vi "Add Icon From Path.vi"(7 "Icon Index (Next)":i32=-1, 8 "error in (no error)":errorcluster, 9 "Icon Name":string, 10 "Image Path":path, 11 "Toolbar Control in":refnum<class "Toolbar Control.lvclass">) -> (0 "error out":errorcluster, 3 "Toolbar Control out":refnum<class "Toolbar Control.lvclass">)   [LabVIEW 2011, in "Toolbar Control.lvclass"]
doc: "This VI will add the image <B>Image Path</B> to the <B>Toolbar Control in</B> at the available location or if specified by <B>Icon Index (Next)</B>. The name of the button will default to the file name or one provided by <B>Icon Name</B>. The image file can be a PNG with alpha layers.\n\n-------------\nDeveloped by Brian Hoover (hooovahh)"
uses:
  Toolbar Control.lvclass
  Toolbar Control.lvclass/Toolbar Control.ctl
  Controls/Icon Data.ctl
  <vilib>/picture/picture.llb/imagedata.ctl
  Controls/Button State.ctl
  Controls/Icon Type.ctl
  <vilib>/Utility/miscctls.llb/LVRectTypeDef.ctl
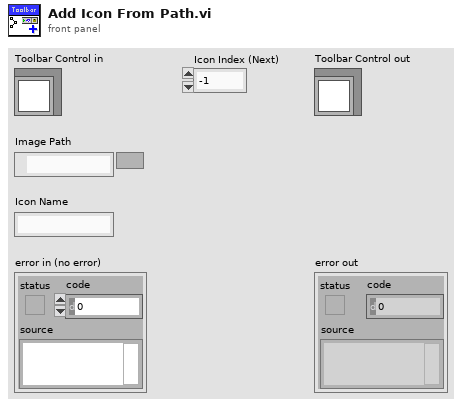
[diagram p1: front panel]
types:
  T1 = typedef "LVRectTypeDef.ctl" = cluster{"Left":i16, "Top":i16, "Right":i16, "Bottom":i16}
  T2 = typedef "Toolbar Control.lvclass/Icon Data.ctl" = cluster{"Original Image Path":path, "Original Image Data":T3, "Scaled Icon":picture, "Button Name":string, "Button State":T4, "Icon Type":T5}
  T3 = typedef "imagedata.ctl" = cluster{"image type":i32, "image depth":i32, "image":u8[], "mask":u8[], "colors":u32[], "Rectangle":cluster{"left":i16, "top":i16, "right":i16, "bottom":i16}}
  T4 = typedef "Toolbar Control.lvclass/Button State.ctl" = enum8{"Enabled", "Disabled", "Disabled and Grayed Out"}
  T5 = typedef "Icon Type.ctl" = enum16{"Normal Icon", "Separator Icon", "More Options"}
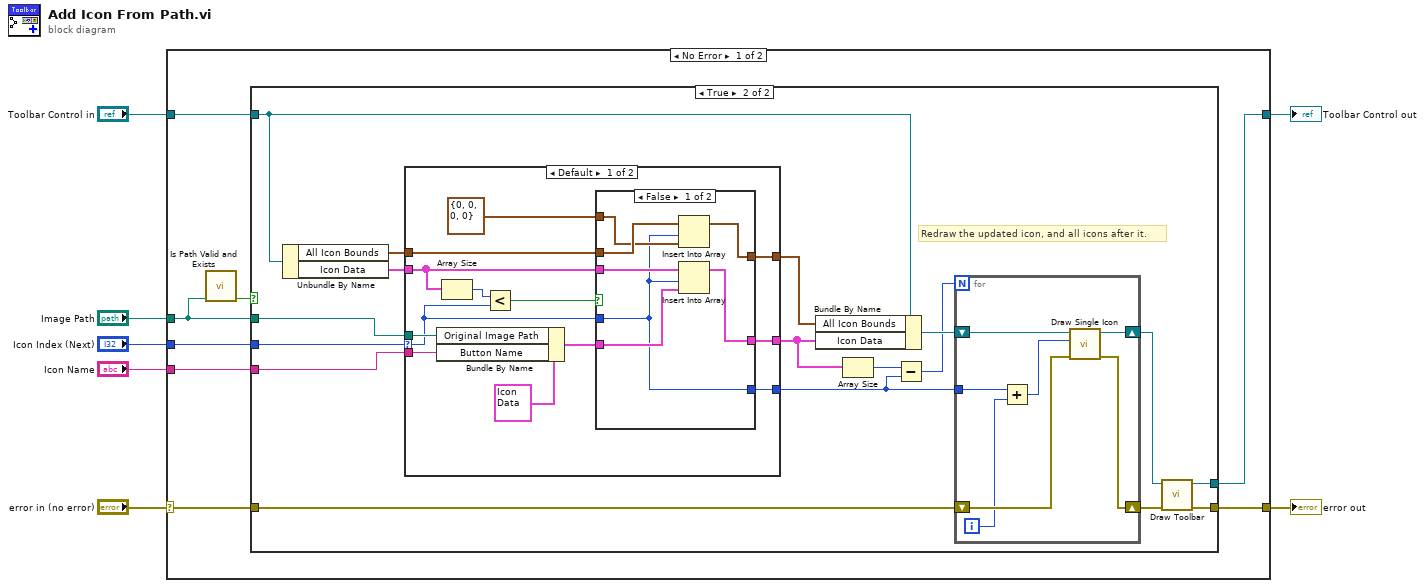
[diagram p0: block diagram]
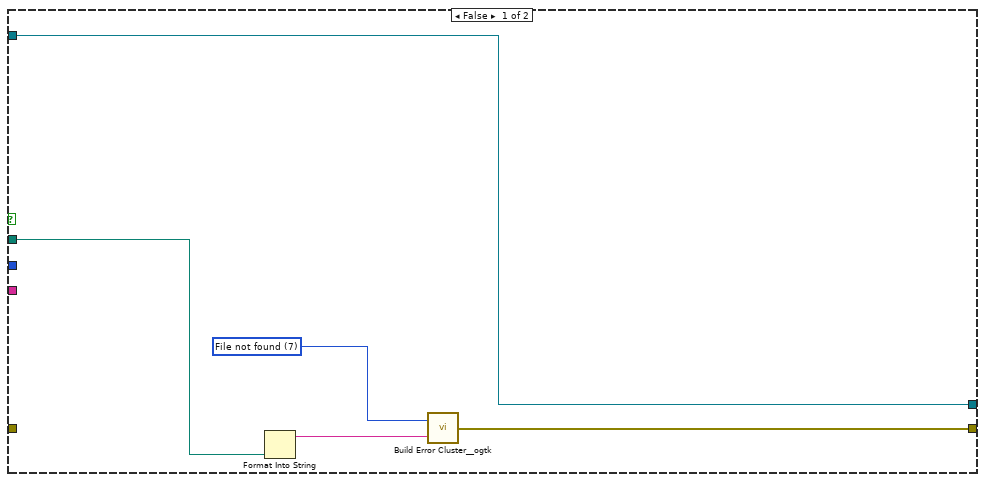
[diagram p2: hidden frame]
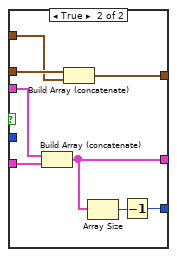
[diagram p3: hidden frame]
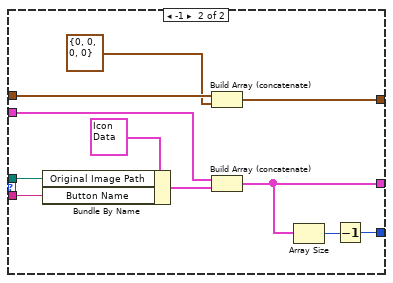
[diagram p4: hidden frame]
diagram:
  n1 = case shown="No Error" "error in (no error)" {
    selector: "error in (no error)" -> [w12 w85]
    tunnel: [w11 w85] -> w6
    tunnel: [w10 w84] -> w4
    tunnel: "Toolbar Control in" -> [w15 w84]
    tunnel: "Image Path" -> [w9 _]
    tunnel: "Icon Index (Next)" -> [w14 _]
    tunnel: "Icon Name" -> [w13 _]
    frame No Error {
      n2 = call "Is Path Valid and Exists.vi"("File/Folder Path"=w9) -> ("Valid and Exists?"=w8:bool)  [unwired: 9 in, 1 out]
      n3 = case shown="True" w8 {
        tunnel: w15 -> [w20 w37]
        tunnel: w14 -> [_ w35]
        tunnel: w13 -> [_ w34]
        tunnel: w12 -> [_ w32]
        tunnel: [w19 w23] -> w11
        tunnel: [w20 w22] -> w10
        tunnel: w9 -> [w17 w21]
        frame False {
          w18 = 7 items=["No error", "Argument error", "Memory is full", "Out of zone", "End of file", "File already open", "Generic file I/O error", "File not found", "File permission error", "Disk is full", "Duplicate path", "Too many files open", "System feature not enabled", "Resource file not found", "Cannot add resource", "Resource not found", "Image not found", "Image memory error", "Pen does not exist", "Config type invalid", "Config token not found", "Config parse error", "Config memory error", "Bad external code format", "Bad external code offset", "External code not present", "Null window", "Destroy window error", "Null menu", "Print aborted", "Bad print record", "Print driver error", "Windows error during printing", "Memory error during printing", "Print dialog error", "Generic print error", "Invalid device refnum", "Device not found", "Device parameter error", "Device unit error", "Cannot open device", "Device call aborted", "Generic error", "Cancelled by user", "Object ID too low", "Object ID too high", "Object not in heap", "Unknown heap", "Unknown object (invalid DefProc)", "Unknown object (DefProc not in table)", "Message out of range", "Invalid (null) method", "Unknown message", "Manager call not supported", "Bad address", "Network operation in progress", "Network operation timed out", "Connection is busy", "Network attribute not supported", "Network error", "Address in use", "System out of memory", "Connection aborted", "Connection refused", "Not connected", "Already connected", "Connection closed", "Initialization error (interapplication manager)", "Bad occurrence", "Wait on unbound occurrence handler", "Occurrence queue overflow", "Datalog type conflict", "Unused", "Unrecognized type (interapplication manager)", "Memory corrupt", "Failed to make temporary DLL", "Old CIN version", "Drag socket not found", "Failed to load drop-object", "Failed to register OLE object", "Failed to release OLE object", "Format specifier type mismatch", "Unknown format specifier", "Too few format specifiers", "Too many format specifiers", "Scan failed", "Newer CIN version", "Error converting to variant", "Runtime menu error", "Password tampered", "Variant attribute not found", "Incompatible variant data type", "Event data is not available", "Event Store is not present", "Occurrence is not found", "Event Queue is not created", "Event info is not available", "Refnum passed is NULL", "Error retrieving Class GUID", "Error retrieving CoClass GUID", "Error retrieving TypeLib GUID.", "Bad built application magic bytes.", "Specific driver is different from the specific driver associated with the Logical Name.", "There is no session opened to the class driver.", "Max Error", "MAX - Error with config objects", "MAX - Error loading configuration", "MAX - Group not supported"]
          n4 = Format Into String(w17) -> (resulting string=w16:string)  [unwired: 3 in, 1 out]
          n5 = call <userlib>:"Build Error Cluster__ogtk.vi"("String to Prepend to source (\"\")"=w16, "code"=w18) -> ("error out"=w19:errorcluster)
        }
        frame True {
          # "Redraw the updated icon, and all icons after it."
          n6 = Unbundle By Name(w37) -> ("All Icon Bounds"=w31:T1[], "Icon Data"=w36:T2[])
          n7 = case shown="Default" w35 {
            selector: w35 -> [w49 _]
            tunnel: w21 -> [w57 w82]
            tunnel: w34 -> [w56 w81]
            tunnel: w36 -> [w54 w80]
            tunnel: [w50 w78] -> w29
            tunnel: [w48 w76] -> w27
            tunnel: w31 -> [w47 w75]
            tunnel: [w46 w73] -> w30
            frame Default {
              n8 = Bundle By Name(cluster=T2 {"Original Image Path"=path "", "Original Image Data"={"image type"=0, "image depth"=0, "image"=[], "mask"=[], "colors"=[], "Rectangle"={"left"=0, "top"=0, "right"=0, "bottom"=0}}, "Scaled Icon"=bytes[0], "Button Name"="", "Button State"=enum."Enabled", "Icon Type"=enum."Normal Icon"} ("Cluster"), "Original Image Path"=w57, "Button Name"=w56) -> (w51:T2)
              n9 = Array Size(array=w54) -> (size(s)=w53:i32)
              n10 = Less?(x=w53, y=w49) -> (x < y?=w52:bool)
              n11 = case shown="False" w52 {
                tunnel: w54 -> [w64 w72]
                tunnel: w51 -> [w63 w71]
                tunnel: [w62 w69] -> w50
                tunnel: w49 -> [w58 _]
                tunnel: [w58 w68] -> w48
                tunnel: w47 -> [w61 w67]
                tunnel: [w60 w66] -> w46
                tunnel: T1 {"Left"=0, "Top"=0, "Right"=0, "Bottom"=0} ("Icon Bounds") -> [w59 w65]
                frame False {
                  n12 = Insert Into Array(array=w61, index=w58, new element=w59) -> (w60:T1[])
                  n13 = Insert Into Array(array=w64, index=w58, new element=w63) -> (w62:T2[])
                }
                frame True {
                  n14 = Build Array (concatenate)(w72, w71) -> (w69:T2[])
                  n15 = Build Array (concatenate)(w67, w65) -> (w66:T1[])
                  n16 = Array Size(array=w69) -> (size(s)=w70:i32)
                  n17 = Decrement(x=w70) -> (x-1=w68:i32)
                }
              }
            }
            frame -1 {
              n18 = Bundle By Name(cluster=T2 {"Original Image Path"=path "", "Original Image Data"={"image type"=0, "image depth"=0, "image"=[], "mask"=[], "colors"=[], "Rectangle"={"left"=0, "top"=0, "right"=0, "bottom"=0}}, "Scaled Icon"=bytes[0], "Button Name"="", "Button State"=enum."Enabled", "Icon Type"=enum."Normal Icon"} ("Cluster"), "Original Image Path"=w82, "Button Name"=w81) -> (w79:T2)
              n19 = Build Array (concatenate)(w75, T1 {"Left"=0, "Top"=0, "Right"=0, "Bottom"=0} ("Icon Bounds")) -> (w73:T1[])
              n20 = Build Array (concatenate)(w80, w79) -> (w78:T2[])
              n21 = Array Size(array=w78) -> (size(s)=w77:i32)
              n22 = Decrement(x=w77) -> (x-1=w76:i32)
            }
          }
          n23 = Bundle By Name(cluster=w37, "All Icon Bounds"=w30, "Icon Data"=w29) -> (w33:refnum<class "Toolbar Control.lvclass">)
          n24 = Array Size(array=w29) -> (size(s)=w28:i32)
          n25 = Subtract(x=w28, y=w27) -> (x-y=w26:i32)
          n26 = for {
            N: w26 -> [_]
            tunnel: w27 -> [w40]
            shift-right: [w43] -> w25
            shift-left: w33 -> [w44]
            shift-right: [w41] -> w24
            shift-left: w32 -> [w42]
            i -> [w39]
            n27 = Add(x=w40, y=w39) -> (x+y=w38:i32)
            n28 = call "Draw Single Icon.vi"("error in (no error)"=w42, "Icon Index"=w38, "Toolbar Control in"=w44) -> ("error out"=w41:errorcluster, "Toolbar Control out"=w43:refnum<class "Toolbar Control.lvclass">)  [unwired: 7 in]
          }
          n29 = call "Draw Toolbar.vi"("error in (no error)"=w24, "Toolbar Control in"=w25) -> ("error out"=w23:errorcluster, "Toolbar Control out"=w22:refnum<class "Toolbar Control.lvclass">)  [unwired: 7 in, 1 out]
        }
      }
    }
    frame Error {
    }
  }
  "error out" <- w6
  "Toolbar Control out" <- w4
